vi "Messung_Hystereseschleife.vi"(7 "Messung Hystereseschleife":T3, 8 "Error in":errorcluster caption="Error_in", 9 "Globale Variablen":T1, 10 "GUI data":T4={"Eisenquerschnitt [mm^2]"=45.0, "Wirksame Länge [cm]"=94.0, "Primärwindungszahl"=700.0, "Sekundärwindungszahl"=700.0, "Messwiderstand [Ohm]"=1.0, "Spannungsteilerverhaeltnis (1/x)"=1.0, "Probenbezeichnung"="", "Dichte des Eisens [g/cm^3]"=7.0, "magn. Flussdichte [T]"=2.0, "Frequenz [Hz]"=50.0, "Namen"="", "Gruppe"=""}, 11 "GUI Einstellungen":T2) -> (0 "Error out":errorcluster caption="Error_out", 1 "Globale Variablen out":T1, 2 "GUI data out":T4, 3 "GUI Einstellungen out":T2, 5 "Messung Hystereseschleife out":T3)   [LabVIEW 2016]
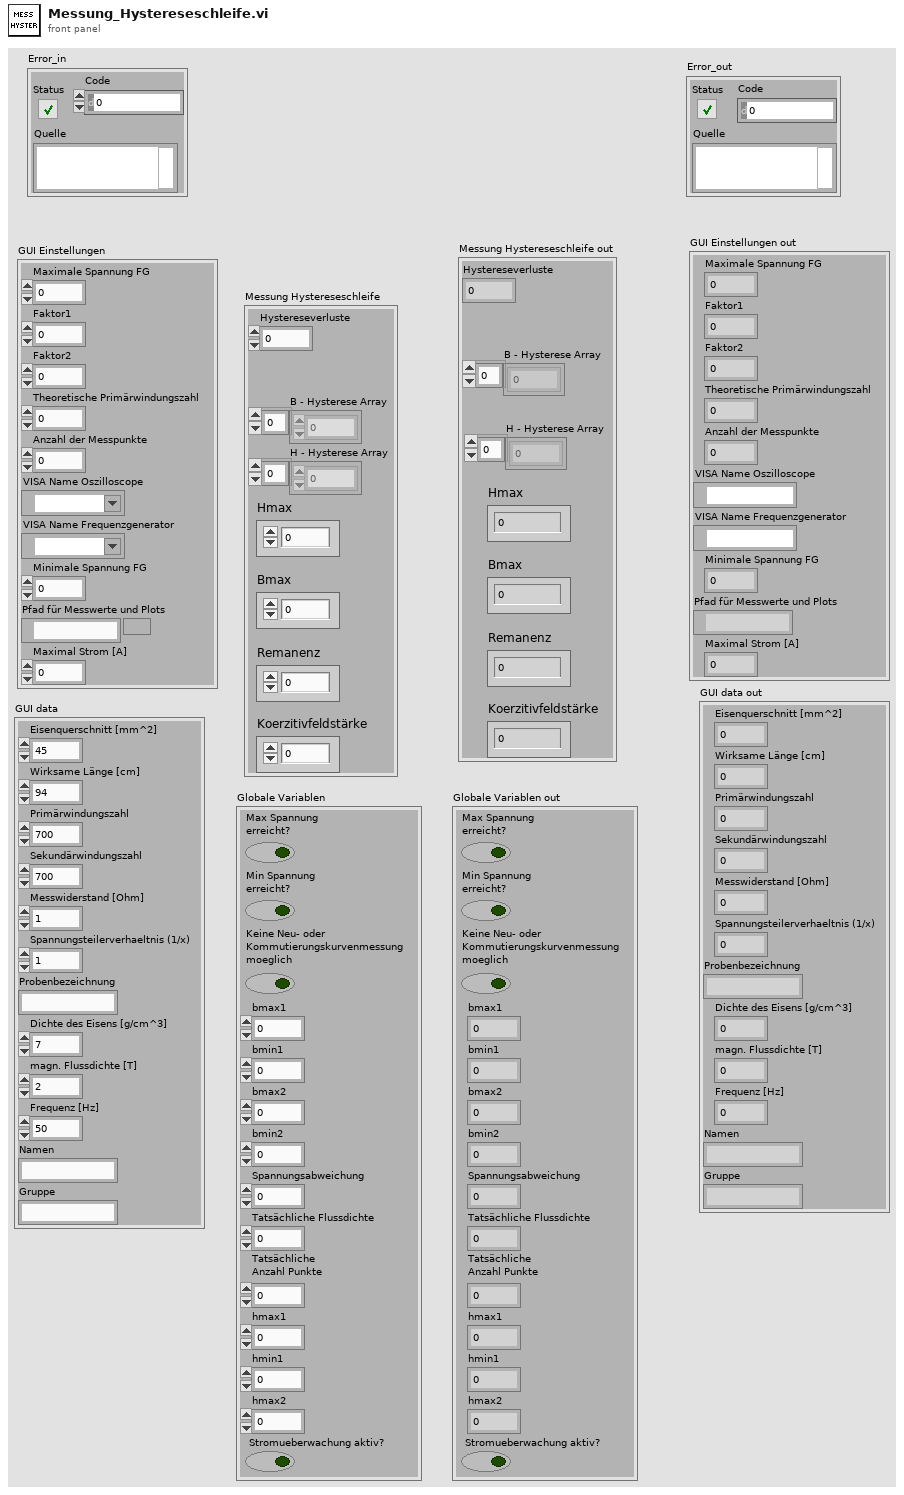
[diagram p1: front panel]
types:
  T1 = cluster{"Max Spannung\nerreicht?":bool, "Min Spannung\nerreicht?":bool, "Keine Neu- oder\nKommutierungskurvenmessung\nmoeglich":bool, "bmax1":dbl, "bmin1":dbl, "bmax2":dbl, "bmin2":dbl, "Spannungsabweichung":dbl, "Tatsächliche Flussdichte":dbl, "Tatsächliche \nAnzahl Punkte":dbl, "hmax1":dbl, "hmin1":dbl, "hmax2":dbl, " Stromueberwachung aktiv?":bool}
  T2 = cluster{"Maximale Spannung FG":dbl, "Faktor1":dbl, "Faktor2":dbl, "Theoretische Primärwindungszahl":dbl, "Anzahl der Messpunkte":i32, "VISA Name Oszilloscope":refnum<visa-resource-name>, "VISA Name Frequenzgenerator":refnum<visa-resource-name>, "Minimale Spannung FG":dbl, "Pfad für Messwerte und Plots":path, "Maximal Strom [A] ":dbl}
  T3 = cluster{"Hystereseverluste":dbl, "B - Hysterese Array":dbl[], "H - Hysterese Array":dbl[], "Hmax":dbl, "Bmax":dbl, "Remanenz":dbl, "Koerzitivfeldstärke":dbl}
  T4 = cluster{"Eisenquerschnitt [mm^2]":dbl, "Wirksame Länge [cm]":dbl, "Primärwindungszahl":dbl, "Sekundärwindungszahl":dbl, "Messwiderstand [Ohm]":dbl, "Spannungsteilerverhaeltnis (1/x)":dbl, "Probenbezeichnung":string, "Dichte des Eisens [g/cm^3]":dbl, "magn. Flussdichte [T]":dbl, "Frequenz [Hz]":dbl, "Namen":string, "Gruppe":string}
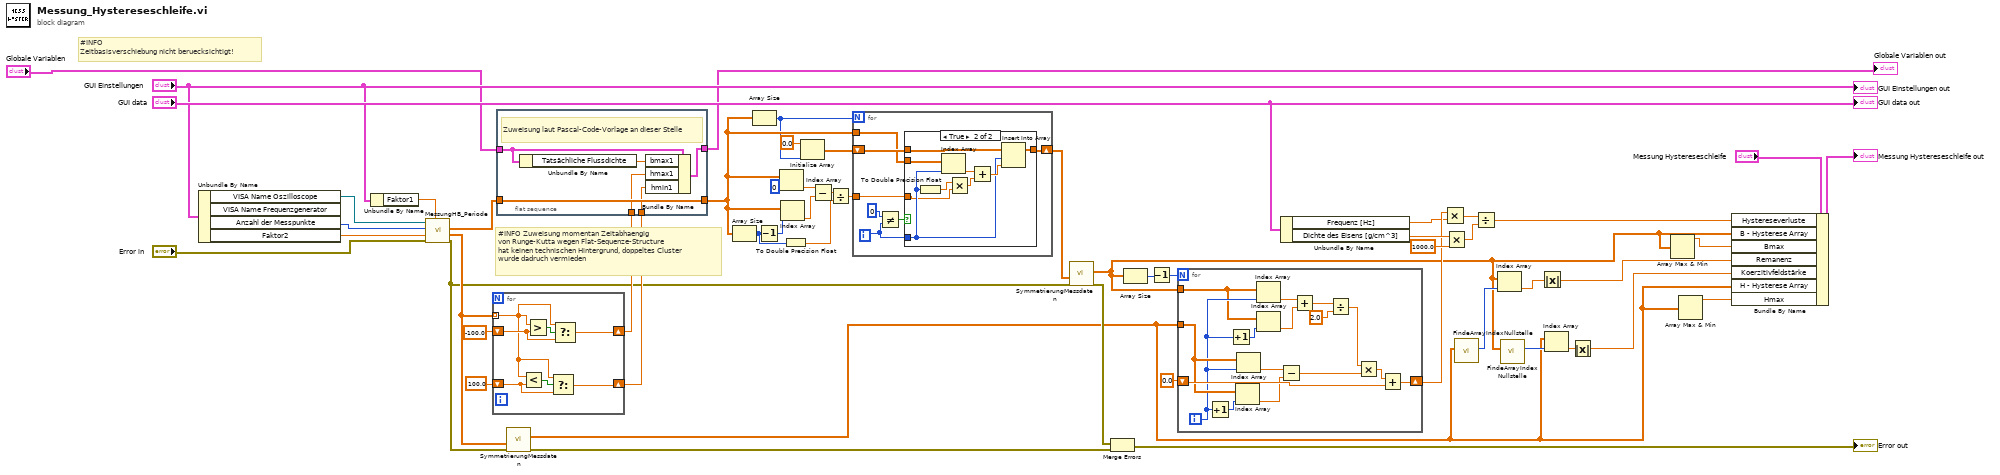
[diagram p0: block diagram]
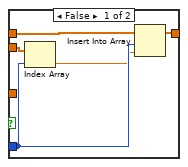
[diagram p2: hidden frame]
diagram:
  # "#INFO\nZeitbasisverschiebung nicht beruecksichtigt!"
  # "#INFO Zuweisung momentan Zeitabhaengig\nvon Runge-Kutta wegen Flat-Sequenze-Structure\nhat keinen technischen Hintergrund, doppeltes Cluster\nwurde dadruch vermieden"
  n1 = Unbundle By Name("GUI Einstellungen") -> ("VISA Name Oszilloscope"=w29:refnum<visa-resource-name>, "Anzahl der Messpunkte"=w28:i32, "Faktor2"=w27:dbl)  [unwired: 1 out]
  n2 = Unbundle By Name("GUI Einstellungen") -> ("Faktor1"=w25:dbl)
  n3 = call "MessungHB_Periode.vi"("Faktor 1"=w25, "Error_in"="Error in", "Faktor2 (1)"=w27, "Anzahl der Messpunkte"=w28, "VISA Name OZ in(OZ)"=w29) -> ("Error_out"=w23:errorcluster, "H-Messdaten einer periode"=w26:dbl[], "B-Messdaten einer periode"=w24:dbl[])  [unwired: 3 in, 1 out]
  n4 = for {
    shift-right: [w60] -> w32
    shift-left: -100.0 -> [w61]
    shift-right: [w57] -> w31
    shift-left: 100.0 -> [w56]
    tunnel: w26 -> [w55] mode=indexing
    n5 = Less?(x=w55, y=w56) -> (x < y?=w58:bool)
    n6 = Greater?(x=w55, y=w61) -> (0:w59:bool)
    n7 = Select(t=w55, s=w58, f=w56) -> (s? t:f=w57:dbl)
    n8 = Select(t=w55, s=w59, f=w61) -> (s? t:f=w60:dbl)
  }
  n9 = flat-sequence {
    tunnel: w24 -> [w67]
    tunnel: [w67] -> w22
    tunnel: "Globale Variablen" -> [w65]
    tunnel: [w66] -> w1
    tunnel: w32 -> [w63]
    tunnel: w31 -> [w62]
    frame #0 {
      # "Zuweisung laut Pascal-Code-Vorlage an dieser Stelle"
      n10 = Unbundle By Name(w65) -> ("Tatsächliche Flussdichte"=w64:dbl)
      n11 = Bundle By Name(cluster=w65, "bmax1"=w64, "hmax1"=w63, "hmin1"=w62) -> (w66:T1)
    }
  }
  n12 = call "SymmetrierungMessdaten.vi"("error in"=w23, "Input Array"=w26) -> ("error out"=w39:errorcluster, "Output Array"=w3:dbl[])  [unwired: 3 in, 3 out]
  n13 = Array Size(array=w22) -> (size(s)=w47:i32)
  n14 = Array Size(array=w22) -> (size(s)=w18:i32)
  n15 = Decrement(x=w47) -> (x-1=w49:i32)
  n16 = Index Array(array=w22, index=0) -> (element=w51:dbl)
  n17 = Index Array(array=w22, index=w49) -> (element=w50:dbl)
  n18 = To Double Precision Float(number=w47) -> (double precision float=w46:dbl)
  n19 = Initialize Array(0.0 ("element"), w18) -> (w20:dbl[])
  n20 = Subtract(x=w51, y=w50) -> (x-y=w48:dbl)
  n21 = Divide(x=w48, y=w46) -> (x/y=w11:dbl)
  n22 = for {
    N: w18 -> [_]
    tunnel: w22 -> [w69]
    shift-right: [w70] -> w21
    shift-left: w20 -> [w71]
    tunnel: w11 -> [w68]
    i -> [w72]
    n23 = Not Equal?(x=0, y=w72) -> (x != y?=w73:bool)
    n24 = case shown="True" w73 {
      tunnel: w71 -> [w78 w88]
      tunnel: w72 -> [w76 w81]
      tunnel: [w79 w87] -> w70
      tunnel: w69 -> [w77 w86]
      tunnel: w68 -> [_ w80]
      frame False {
        n25 = Index Array(array=w77, index=w76) -> (element=w75:dbl)
        n26 = Insert Into Array(array=w78, index=w76, new element=w75) -> (w79:dbl[])
      }
      frame True {
        n27 = To Double Precision Float(number=w81) -> (double precision float=w83:dbl)
        n28 = Index Array(array=w86, index=w81) -> (element=w85:dbl)
        n29 = Multiply(x=w83, y=w80) -> (x*y=w84:dbl)
        n30 = Add(x=w85, y=w84) -> (x+y=w82:dbl)
        n31 = Insert Into Array(array=w88, index=w81, new element=w82) -> (w87:dbl[])
      }
    }
  }
  n32 = call "SymmetrierungMessdaten.vi"("error in"=w23, "Input Array"=w21) -> ("error out"=w10:errorcluster, "Output Array"=w4:dbl[])  [unwired: 3 in, 3 out]
  n33 = Merge Errors(w10, w39) -> (→"Error out":errorcluster)
  n34 = Array Size(array=w4) -> (size(s)=w45:i32)
  n35 = Decrement(x=w45) -> (x-1=w44:i32)
  n36 = for {
    N: w44 -> [_]
    tunnel: w4 -> [w94]
    shift-right: [w103] -> w9
    shift-left: 0.0 -> [w104]
    tunnel: w3 -> [w101]
    i -> [w95]
    n37 = Increment(x=w95) -> (x+1=w100:i32)
    n38 = Increment(x=w95) -> (x+1=w96:i32)
    n39 = Index Array(array=w101, index=w100) -> (element=w99:dbl)
    n40 = Index Array(array=w101, index=w95) -> (element=w102:dbl)
    n41 = Index Array(array=w94, index=w95) -> (element=w97:dbl)
    n42 = Index Array(array=w94, index=w96) -> (element=w93:dbl)
    n43 = Subtract(x=w102, y=w99) -> (x-y=w98:dbl)
    n44 = Add(x=w97, y=w93) -> (x+y=w92:dbl)
    n45 = Divide(x=w92, y=2.0) -> (x/y=w90:dbl)
    n46 = Multiply(x=w90, y=w98) -> (x*y=w89:dbl)
    n47 = Add(x=w89, y=w104) -> (x+y=w103:dbl)
  }
  n48 = Unbundle By Name("GUI data") -> ("Frequenz [Hz]"=w8:dbl, "Dichte des Eisens [g/cm^3]"=w36:dbl)
  n49 = Multiply(x=w9, y=w8) -> (x*y=w42:dbl)
  n50 = Multiply(x=w36, y=1000.0) -> (x*y=w40:dbl)
  n51 = call "FindeArrayIndexNullstelle.vi"("Array"=w3) -> ("Array Index Nullstelle"=w7:i32)  [unwired: 10 in]
  n52 = Divide(x=w42, y=w40) -> (x/y=w33:dbl)
  n53 = Index Array(array=w4, index=w7) -> (element=w14:dbl)
  n54 = call "FindeArrayIndexNullstelle.vi"("Array"=w4) -> ("Array Index Nullstelle"=w6:i32)  [unwired: 10 in]
  n55 = Absolute Value(x=w14) -> (abs(x)=w5:dbl)
  n56 = Index Array(array=w3, index=w6) -> (element=w13:dbl)
  n57 = Absolute Value(x=w13) -> (abs(x)=w12:dbl)
  n58 = Array Max & Min(array=w4) -> (max value=w15:dbl)  [unwired: 3 out]
  n59 = Array Max & Min(array=w3) -> (max value=w16:dbl)  [unwired: 3 out]
  n60 = Bundle By Name(cluster="Messung Hystereseschleife", "Hystereseverluste"=w33, "B - Hysterese Array"=w4, "Bmax"=w15, "Remanenz"=w5, "Koerzitivfeldstärke"=w12, "H - Hysterese Array"=w3, "Hmax"=w16) -> (→"Messung Hystereseschleife out":T3)
  "GUI data out" <- "GUI data"
  "GUI Einstellungen out" <- "GUI Einstellungen"
  "Globale Variablen out" <- w1
